vi "Get Pot Refnum.vi"(10 "Side":enum16{"Left", "Right"}(ring), 11 "arm in":refnum<class "arm.lvclass">) -> (2 "PotDevRef":T1={"DevStatus"={"status"=FALSE, "code"=0, "source"=""}, "Analog Channel"=enum."Invalid", "Invert Output"=FALSE}, 3 "arm out":refnum<class "arm.lvclass">)   [LabVIEW 2015, in "arm.lvclass"]
uses:
  arm.lvclass
  <vilib>/Rock Robotics/WPI/Potentiometer/WPI_PotentiometerDevRef.ctl
  <vilib>/Rock Robotics/SystemInterfaces/AI/FPGA_AIChannel.ctl
  arm.lvclass/arm.ctl
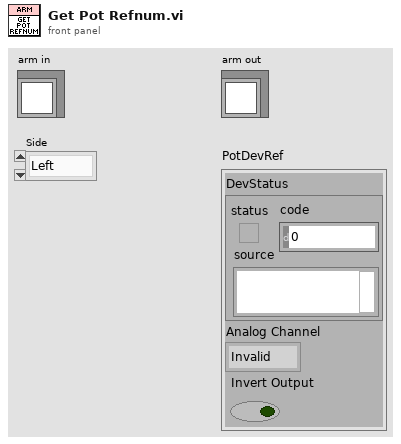
[diagram p1: front panel]
types:
  T1 = typedef "WPI_PotentiometerDevRef.ctl" = cluster{"DevStatus":errorcluster, "Analog Channel":T2, "Invert Output":bool}
  T2 = typedef "FPGA_AIChannel.ctl" = enum8{"AI 0", "AI 1", "AI 2", "AI 3", "AI MXP 0", "AI MXP 1", "AI MXP 2", "AI MXP 3", "Invalid"}
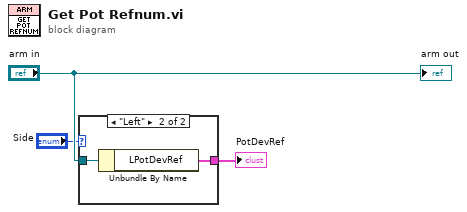
[diagram p0: block diagram]
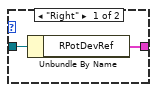
[diagram p2: hidden frame]
diagram:
  n1 = case shown="\"Left\"" "Side" {
    tunnel: "arm in" -> [w5 w7]
    tunnel: [w4 w6] -> w2
    frame "Right" {
      n2 = Unbundle By Name(w5) -> ("RPotDevRef"=w4:T1)
    }
    frame "Left" {
      n3 = Unbundle By Name(w7) -> ("LPotDevRef"=w6:T1)
    }
  }
  "PotDevRef" <- w2
  "arm out" <- "arm in"
